vi "Get Audit Trail Data.vi"(8 "error in (no error)":errorcluster, 9 "connection reference":T1, 10 "To":timestamp, 11 "From":timestamp) -> (0 "error out":errorcluster, 3 "data":string[][](array[string]))   [LabVIEW 2018]
uses:
  <vilib>/addons/database/Connection.llb/Conn ObjectReference.ctl
  Controls/SQL Date Time Format Specifier.ctl
  <vilib>/addons/database/_DB Variant To Data/Database Variant To Data.xnode
  <vilib>/addons/database/NI_Database_API.lvlib
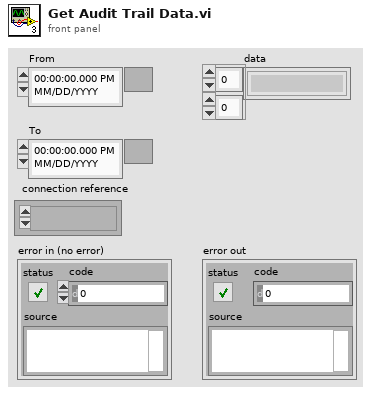
[diagram p1: front panel]
types:
  T1 = typedef "NI_Database_API.lvlib/Conn ObjectReference.ctl" = refnum<k1>
  T2 = typedef "SQL Date Time Format Specifier.ctl" = string
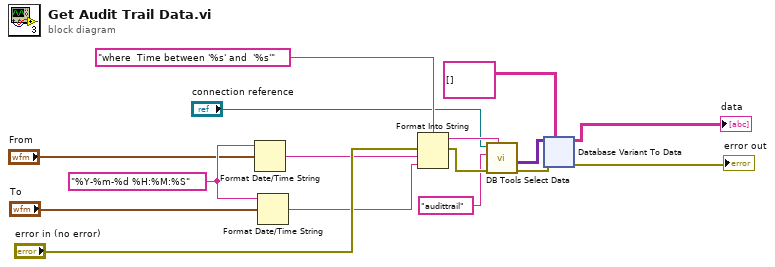
[diagram p0: block diagram]
diagram:
  w3 = T2 "%Y-%m-%d %H:%M:%S" ("time format string (%c)")
  n1 = Format Date/Time String(time format string (%c)=w3, seconds (now)="From") -> (date/time string=w6:string)  [unwired: 1 in]
  n2 = Format Date/Time String(time format string (%c)=w3, seconds (now)="To") -> (date/time string=w7:string)  [unwired: 1 in]
  n3 = Format Into String(format string="where  Time between '%s' and  '%s'", error in="error in (no error)", w6, w7) -> (resulting string=w8:string, error out=w15:errorcluster)  [unwired: 1 in]
  n4 = call <vilib>:"DB Tools Select Data.vi"("condition"=w8, "error in (no error)"=w15, "table"="audittrail", "connection reference"="connection reference") -> ("error out"=w10:errorcluster, "data"=w11:variant[][])  [unwired: 2 in, 1 out]
  n5 = xnode "Database Variant To Data"("database variant"=w11, "error in (no error)"=w10, "type"=string[][] []) -> ("data"=→"data":string[][], "error out"=→"error out":errorcluster)
